vi "str to certification path.vi"(4 "node text":string) -> (1 "File Path Control":path)   [LabVIEW 2013, in "OPCUA XML.lvlib"]
uses:
  OPCUA XML.lvlib
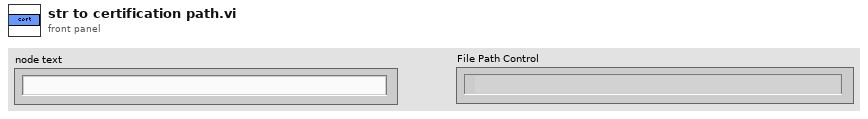
[diagram p1: front panel]
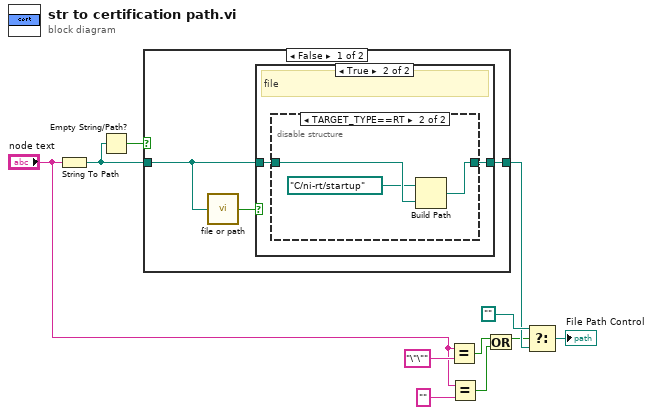
[diagram p0: block diagram]
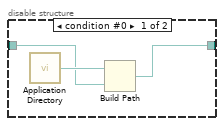
[diagram p3: hidden frame]
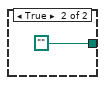
[diagram p4: hidden frame]
diagram:
  n1 = String To Path(string="node text") -> (path=w10:path)
  n2 = Empty String/Path?(string/path=w10) -> (empty?=w11:bool)
  n3 = case shown="False" w11 {
    tunnel: [w13 path ""] -> w7
    tunnel: w10 -> [w12 _]
    frame False {
      n4 = call "file or path.vi"("Path"=w12) -> ("file/path&file"=w14:bool)  [unwired: 2 in]
      n5 = case shown="True" w14 {
        tunnel: [w15 w16] -> w13
        tunnel: w12 -> [w15 w17]
        frame False {
          # "path"
        }
        frame True {
          # "file"
          n6 = disable-structure shown="TARGET_TYPE==RT" {
            disable-tunnel: w17 -> [w19 w22]
            disable-tunnel: [w18 w23] -> w16
            frame condition #0 {
              n7 = call <vilib>:"Application Directory.vi"() -> ("Application Directory"=w20:path)
              n8 = Build Path(base path=w20, name or relative path=w19) -> (appended path=w18:path)
            }
            frame condition #1 (active) {
              n9 = Build Path(base path=path "C:/ni-rt/startup", name or relative path=w22) -> (appended path=w23:path)
            }
          }
        }
      }
    }
    frame True {
    }
  }
  n10 = Equal?(x="node text", y="\"\"" ("node text")) -> (x = y?=w2:bool)
  n11 = Equal?(x="node text", y="" ("node text")) -> (x = y?=w1:bool)
  n12 = Or(x=w2, y=w1) -> (x .or. y?=w3:bool)
  n13 = Select(t=path "", s=w3, f=w7) -> (s? t:f=→"File Path Control":path)
